vi "LoadScannedNodes.vi"() -> (3 "Previously Scanned Nodes":T1 {"Year" format="%02d"; "Patient Number" format="%03d"; "Node Number" format="%02d"})   [LabVIEW 2022 SP3]
uses:
  ScannedNodeArray.ctl
  LymphNodeInfo.ctl
  TissueTypeScan.ctl
  PatientGlobals.vi
  <vilib>/Utility/xml.llb/Read From XML File(string).vi
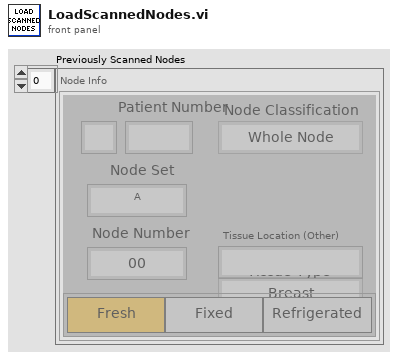
[diagram p1: front panel]
types:
  T1 = typedef "ScannedNodeArray.ctl" = T2[]
  T2 = typedef "LymphNodeInfo.ctl" = cluster{"Patient Number":u32, "Node Set":string, "Node Number":u32, "Tissue Type":T3, "Tissue Location (Other)":string, "Node Classification":enum16{"Whole Node", "Piece A", "Piece B", "Piece C"}, "Fresh?":enum32{"Fresh?", "Fixed?", "Refrigerated?"}, "Year":u32}
  T3 = typedef "TissueTypeScan.ctl" = enum16{"Breast", "Gastric", "Stomach", "Rectal", "Colon", "Head & Neck", "Other"}
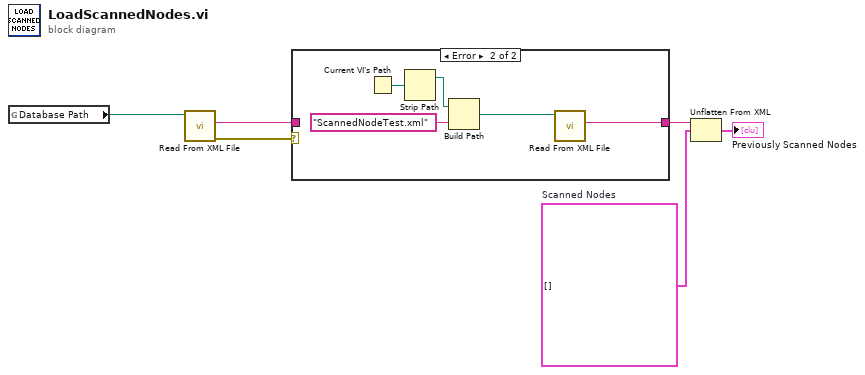
[diagram p0: block diagram]
diagram:
  w6 = T1 []  # Scanned Nodes
  n1 = global read "PatientGlobals.vi" "Database Path"() -> (w4:path)
  n2 = call-poly <vilib>:"Read From XML File.vi"("XML File Path"=w4) -> ("error out"=w3:errorcluster, "XML Elements"=w1:string)  [unwired: 8 in, 1 out]
  n3 = case shown="Error" w3 {
    tunnel: [w7 w12] -> w2
    tunnel: w1 -> [w7 _]
    frame No Error {
    }
    frame Error {
      n4 = Current VI's Path() -> (path=w11:path)
      n5 = Strip Path(path=w11) -> (stripped path=w10:path)  [unwired: 1 out]
      n6 = Build Path(base path=w10, name or relative path="ScannedNodeTest.xml") -> (appended path=w9:path)
      n7 = call-poly <vilib>:"Read From XML File.vi"("XML File Path"=w9) -> ("XML Elements"=w12:string)  [unwired: 8 in, 2 out]
    }
  }
  n8 = Unflatten From XML(xml string=w2, type=w6) -> (value=→"Previously Scanned Nodes":T1)  [unwired: 1 in, 1 out]
